vi "truePosition.vi"() -> ()   [LabVIEW 2009]
panel:
  out "TruePosition":dbl
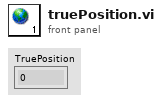
[diagram p1: front panel]
diagram:
